vi "ACQ analog read values.vi"(7 "samples per channel":i32, 8 "error in (no error)":errorcluster, 11 "Tasks ref in":T1) -> (0 "error out":errorcluster, 2 "data":waveform(dbl)[](array[waveform]), 3 "Tasks ref out":T1)   [LabVIEW 2013]
uses:
  Kontrolki/KartaDAQ/ACQ all read tasks.ctl
  <vilib>/DAQmx/read.llb/DAQmx Read (Analog 1D Wfm NChan NSamp).vi
  <vilib>/DAQmx/miscellaneous.llb/DAQmx Fill In Error Info.vi
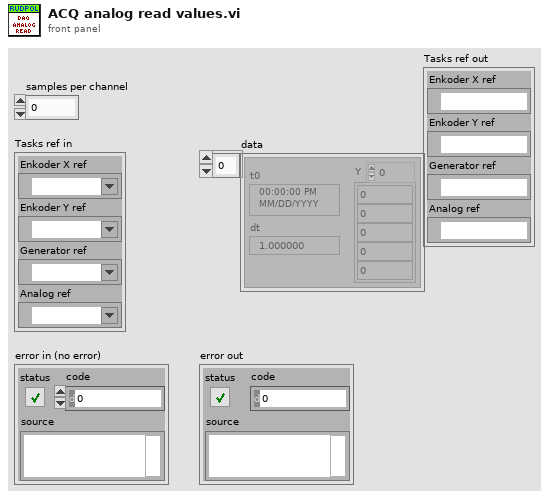
[diagram p1: front panel]
types:
  T1 = typedef "ACQ all read tasks.ctl" = cluster{"Enkoder X ref":refnum<k21>, "Enkoder Y ref":refnum<k21>, "Generator ref":refnum<k21>, "Analog ref":refnum<k21>}
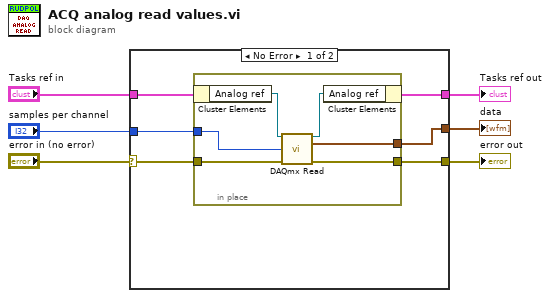
[diagram p0: block diagram]
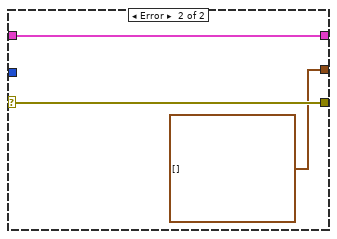
[diagram p2: hidden frame]
diagram:
  n1 = case shown="No Error" "error in (no error)" {
    selector: "error in (no error)" -> [w8 w21]
    tunnel: [w10 waveform(dbl)[] [] ("data")] -> w6
    tunnel: "samples per channel" -> [w7 _]
    tunnel: [w9 w21] -> w4
    tunnel: "Tasks ref in" -> [w12 w20]
    tunnel: [w11 w20] -> w2
    frame No Error {
      n2 = in-place {
        in-place-border: [w16] -> w10
        in-place-border: [w15] -> w9
        in-place-border: w8 -> [w14]
        in-place-border: w7 -> [w13]
        n3 = in-place-cluster #1(w12) -> ("Analog ref"=w18:refnum<k21>)
        n4 = call-poly <vilib>:"DAQmx Read.vi"("task/channels in"=w18, "number of samples per channel"=w13, "error in"=w14) -> ("task out"=w17:refnum<k21>, "data"=w16:waveform(dbl)[], "error out"=w15:errorcluster)  [unwired: 10 in]
        n5 = in-place-cluster #1("Analog ref"=w17) -> (w11:T1)
      }
    }
    frame Error {
    }
  }
  "data" <- w6
  "error out" <- w4
  "Tasks ref out" <- w2
